vi "convert_labview_files.vi"() -> ()   [LabVIEW 2013]
uses:
  Public API/Signal.ctl
  Controls/Role ID.ctl
  Controls/Hardware ID.ctl
  <userlib>/_OpenG.lib/array/array.llb/Search 1D Array (String)__ogtk.vi
  <userlib>/_OpenG.lib/array/array.llb/Delete Elements from 1D Array (String)__ogtk.vi
  <vilib>/addons/database/Connection.llb/Conn Execute.vi
  <vilib>/addons/database/Recordset.llb/Rec Destroy - Connection.vi
  <vilib>/addons/database/NI_Database_API.lvlib
panel:
  in  "Small?":bool
  out "error out":errorcluster
  in  "error in (no error)":errorcluster
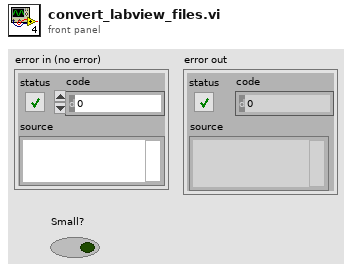
[diagram p1: front panel]
types:
  T1 = typedef "Signal.ctl" = cluster{"Signal ID":i64, "Time Stamp":timestamp, "Dust Event ID":i64, "Role ID":T2, "Data":sgl[], "Signal Length":i32, "dt":sgl, "Offset":dbl, "Hardware ID":T3}
  T2 = typedef "Role ID.ctl" = enum16{"First_Detector", "Second_Detector", "Third_Detector", "LeCroy_CH1", "LeCroy_CH2", "LeCroy_CH3", "LeCroy_CH4", "PSU"}
  T3 = typedef "Hardware ID.ctl" = enum16{"Unknown", "CSA 1", "CSA 2", "CSA 3", "CSA 4", "CSA 5", "CSA 6"}
  T4 = typedef "File Info Record__ogtk.ctl" = cluster{"type":string, "creator":string, "permissions":i32, "data size":i32, "res size":i32, "creation date":u32, "modification date":u32, "bFolder":bool, "bInvisible":bool, "location":cluster{"vertical":i16, "horizontal":i16}, "owner":string, "group":string}
  T5 = typedef "NI_Database_API.lvlib/Conn ObjectReference.ctl" = refnum<k1>
  T6 = typedef "NI_Database_API.lvlib/Rec ObjectReference.ctl" = refnum<k1>
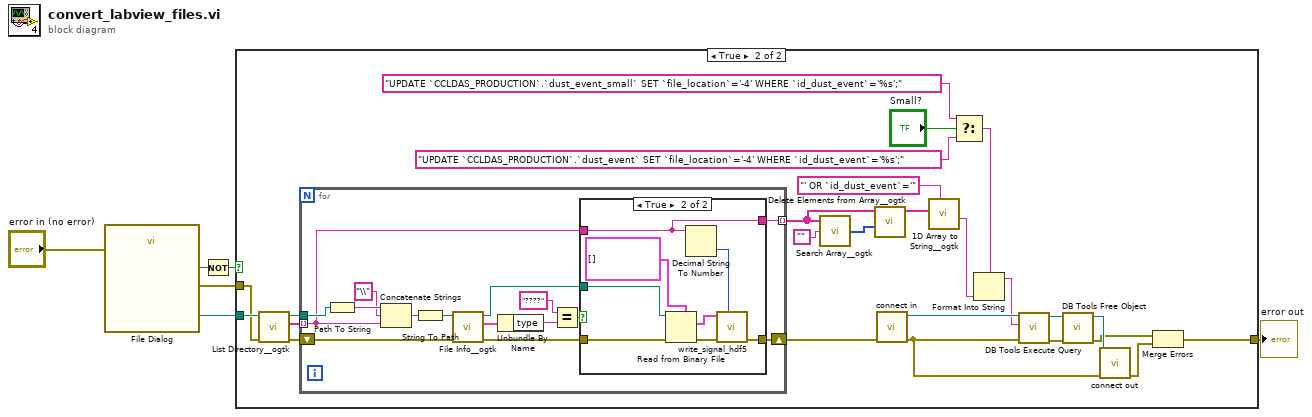
[diagram p0: block diagram]
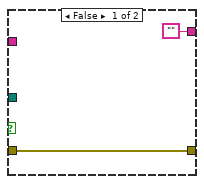
[diagram p3: hidden frame]
diagram:
  n1 = call "File Dialog"("error in"="error in (no error)") -> ("selected path"=w4:path, "cancelled"=w6:bool, "error out"=w3:errorcluster)  [unwired: 11 in, 1 out]
  n2 = Not(x=w6) -> (.not. x?=w5:bool)
  n3 = case shown="True" w5 {
    tunnel: w4 -> [_ w32]
    tunnel: w3 -> [w7 w29]
    tunnel: [w7 w16] -> w1
    frame False {
    }
    frame True {
      n4 = call <userlib>:"List Directory__ogtk.vi"("error in (no error)"=w29, "directory path"=w32) -> ("error out"=w28:errorcluster, "file names"=w31:string[], "dup directory path"=w30:path)  [unwired: 2 in, 1 out]
      n5 = for {
        tunnel: w31 -> [w34] mode=indexing
        tunnel: w30 -> [w46]
        shift-right: [w37] -> w13
        shift-left: w28 -> [w40]
        tunnel: [w33] -> w24 mode=indexing
        n6 = Path To String(path=w46) -> (string=w45:string)
        n7 = Concatenate Strings(w45, "\\" ("string"), w34) -> (w43:string)
        n8 = String To Path(string=w43) -> (path=w42:path)
        n9 = call <userlib>:"File Info__ogtk.vi"("error in (no error)"=w40, "file"=w42) -> ("error out"=w36:errorcluster, "file info"=w47:T4, "file out"=w35:path)  [unwired: 4 in]
        n10 = Unbundle By Name(w47) -> ("type"=w41:string)
        n11 = Equal?(x="????", y=w41) -> (x = y?=w38:bool)
        n12 = case shown="True" w38 {
          tunnel: [w49 w54] -> w37
          tunnel: w36 -> [w49 w57]
          tunnel: w35 -> [_ w55]
          tunnel: w34 -> [_ w50]
          tunnel: ["" w50] -> w33
          frame False {
          }
          frame True {
            n13 = Read from Binary File(5:T1[] [] ("Signal array"), 8:w57, 11:w55) -> (0:w56:errorcluster, 2:w52:T1[])  [unwired: 3 in, 2 out]
            n14 = Decimal String To Number(string=w50) -> (number=w51:i32)  [unwired: 2 in, 1 out]
            n15 = call "write_signal_hdf5.vi"("Index"=w51, "error in"=w56, "Signal array"=w52) -> ("error out"=w54:errorcluster)  [unwired: 7 in, 1 out]
          }
        }
      }
      n16 = call-poly <userlib>:"Search Array__ogtk.vi"("Array"=w24, "Element Data"="") -> ("Indices of Elements"=w25:i32[])  [unwired: 7 in]
      n17 = call-poly <userlib>:"Delete Elements from Array__ogtk.vi"("indices"=w25, "array"=w24) -> ("array w/ subset deleted"=w23:string[])  [unwired: 8 in, 1 out]
      n18 = call "connect in.vi"("error in (no error)"=w13) -> ("error out"=w20:errorcluster, "Database Connection"=w27:T5)  [unwired: 6 in, 1 out]
      n19 = call <userlib>:"1D Array to String__ogtk.vi"("delimiter (Tab)"="' OR `id_dust_event`='", "Array of Strings"=w23) -> ("delimited string"=w21:string)  [unwired: 9 in]
      n20 = Select(t="UPDATE `CCLDAS_PRODUCTION`.`dust_event_small` SET `file_location`='-4' WHERE `id_dust_event`='%s';" ("format string"), s="Small?", f="UPDATE `CCLDAS_PRODUCTION`.`dust_event` SET `file_location`='-4' WHERE `id_dust_event`='%s';" ("format string")) -> (s? t:f=w8:string)
      n21 = Format Into String(format string=w8, w21) -> (resulting string=w12:string)  [unwired: 2 in, 1 out]
      n22 = call-poly <vilib>:"DB Tools Execute Query.vi"("error in (no error)"=w20, "SQL query"=w12, "connection reference"=w27) -> ("error out"=w19:errorcluster, "recordset reference"=w18:T6)  [unwired: 5 in]
      n23 = call-poly <vilib>:"DB Tools Free Object.vi"("error in (no error)"=w19, "recordset reference"=w18) -> ("error out"=w14:errorcluster, "connection reference"=w17:T5)  [unwired: 8 in]
      n24 = call "connect out.vi"("error in (no error)"=w20, "connection reference"=w17) -> ("error out"=w15:errorcluster)  [unwired: 9 in]
      n25 = Merge Errors(w14, w15) -> (w16:errorcluster)
    }
  }
  "error out" <- w1
